vi "Multi-nRF24-BME280-Logger-v1.0.0.vi"() -> ()   [LabVIEW 2018]
uses:
  Program Files (x86)/National Instruments/LabVIEW 2018/examples/Instrument IO/Serial/support/Serial - XON-XOFF Characters.ctl
  Program Files (x86)/National Instruments/LabVIEW 2018/examples/Instrument IO/Serial/support/Serial - ASCII Characters.ctl
  Program Files (x86)/National Instruments/LabVIEW 2018/examples/Instrument IO/Serial/support/Serial - Settings.ctl
  <vilib>/Instr/_visa.llb/VISA Configure Serial Port (Instr).vi
panel:
  in  "Start Button":bool
  out "Log String":string
  in  "No. Of Sensor Modules":i32
  out "error out":errorcluster
  in  "VISA resource name":refnum<visa-resource-name>="COM1"
  out "Response":string
  in  "Stop":bool
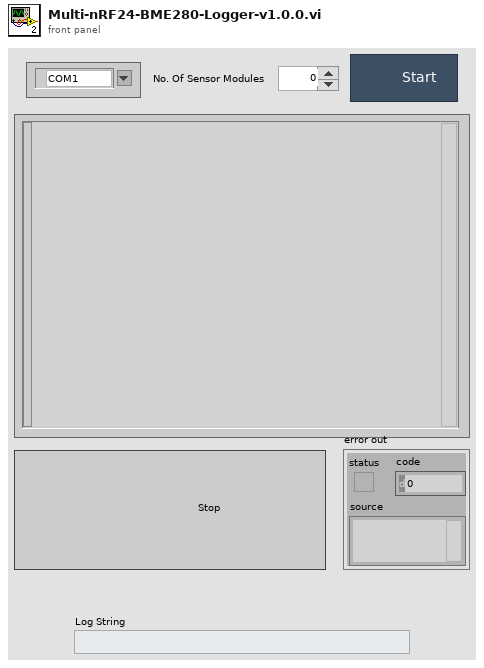
[diagram p1: front panel]
types:
  T1 = typedef "Serial - Settings.ctl" = cluster{"baud rate":u32, "data bits":u16, "parity":enum16{"None", "Odd", "Even", "Mark", "Space"}, "stop bits":u16, "flow control":u16}
  T2 = typedef "Serial - XON-XOFF Characters.ctl" = cluster{"XON":T3, "XOFF":T3}
  T3 = typedef "Serial - ASCII Characters.ctl" = enum16{"NUL", "SOH", "STX", "ETX", "EOT", "ENQ", "ACK", "BEL", "BS", "HT", "LF", "VT", "FF", "CR", "SO", "SI", "DLE", "DC1", "DC2", "DC3", "DC4", "NAK", "SYN", "ETB", "CAN", "EM", "SUB", "ESC", "FS", "GS", "RS", "US", "SP", "!", "\"", "#", "$", "%", "&", "'", "(", ")", "*", "+", ",", "- (-)", ".", "/", "0", "1", "2", "3", "4", "5", "6", "7", "8", "9", ":", ";", "<", "=", ">", "?", "@", "A", "B", "C", "D", "E", "F", "G", "H", "I", "J", "K", "L", "M", "N", "O", "P", "Q", "R", "S", "T", "U", "V", "W", "X", "Y", "Z", "[", "\\", "]", "^", "_", "`", "a", "b", "c", "d", "e", "f", "g", "h", "i", "j", "k", "l", "m", "n", "o", "p", "q", "r", "s", "t", "u", "v", "w", "x", "y", "z", "{", "|", "}", "~"}
  T4 = enum16{"open", "replace", "create", "open or create", "replace or create", "replace or create with confirmation"}
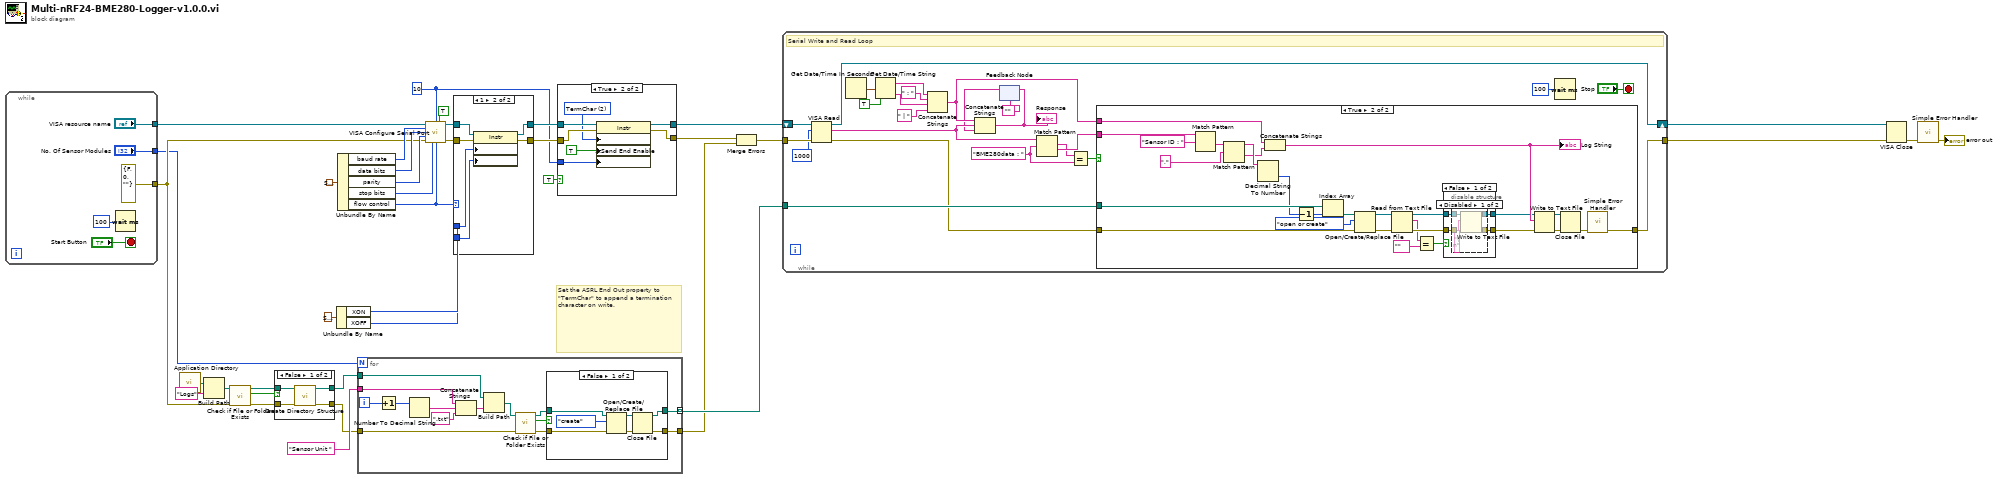
[diagram p0: block diagram]
diagram:
  w8 = u8 10 ("Termination Character")
  # "Set the ASRL End Out property to \"TermChar\" to append a termination character on write."
  n1 = while {
    tunnel: ["No. Of Sensor Modules"] -> w1
    tunnel: ["VISA resource name"] -> w28
    tunnel: [errorcluster {"status"=FALSE, "code"=0, "source"=""} ("error in (no error)")] -> w6
    stop <- "Start Button" stop-if-true
    n2 = Wait (ms)(milliseconds to wait=u32 100) -> ()  [unwired: 1 out]
  }
  n3 = call <vilib>:"Application Directory.vi"() -> ("Application Directory"=w29:path)
  n4 = Build Path(base path=w29, name or relative path="Logs") -> (appended path=w36:path)
  n5 = call <vilib>:"Check if File or Folder Exists.vi"("error in (no error)"=w6, "path"=w36) -> ("error out"=w32:errorcluster, "file or folder exists?"=w34:bool, "dup path"=w33:path)  [unwired: 7 in]
  n6 = case shown="False" w34 {
    tunnel: w33 -> [w46 w48]
    tunnel: w32 -> [w45 w47]
    tunnel: [w44 w48] -> w31
    tunnel: [w43 w47] -> w30
    frame False {
      n7 = call "Create Directory Structure.vi"("error in(no error)"=w45, "Dir Path In"=w46) -> ("error out"=w43:errorcluster, "Dir Path Out"=w44:path)  [unwired: 8 in]
    }
    frame True {
    }
  }
  n8 = Unbundle By Name(T2 {"XON"=enum."DC1", "XOFF"=enum."DC3"} ("XON/XOFF Characters")) -> ("XON"=w14:T3, "XOFF"=w13:T3)
  n9 = Unbundle By Name(T1 {"baud rate"=115200, "data bits"=8, "parity"=enum."None", "stop bits"=10, "flow control"=0} ("Serial Settings")) -> ("baud rate"=w21:u32, "data bits"=w22:u16, "parity"=w23:enum16{"None", "Odd", "Even", "Mark", "Space"}, "stop bits"=w24:u16, "flow control"=w15:u16)
  n10 = for {
    N: w1 -> [_]
    tunnel: "Sensor Unit " ("name or relative path") -> [w60]
    tunnel: w31 -> [w56]
    tunnel: w30 -> [w54]
    tunnel: [w50] -> w5 mode=indexing
    tunnel: [w49] -> w4
    i -> [w62]
    n11 = Increment(x=w62) -> (x+1=w61:i32)
    n12 = Number To Decimal String(number=w61) -> (decimal integer string=w59:string)  [unwired: 1 in]
    n13 = Concatenate Strings(w60, w59, ".txt" ("string")) -> (w57:string)
    n14 = Build Path(base path=w56, name or relative path=w57) -> (appended path=w55:path)
    n15 = call <vilib>:"Check if File or Folder Exists.vi"("error in (no error)"=w54, "path"=w55) -> ("error out"=w51:errorcluster, "file or folder exists?"=w53:bool, "dup path"=w52:path)  [unwired: 7 in]
    n16 = case shown="False" w53 {
      tunnel: w52 -> [w67 w71]
      tunnel: w51 -> [w68 w70]
      tunnel: [w65 w71] -> w50
      tunnel: [w63 w70] -> w49
      frame False {
        n17 = Open/Create/Replace File(file path (use dialog)=w67, error in=w68, operation (0:open)=T4."create") -> (refnum out=w66:refnum<file>, error out=w64:errorcluster)  [unwired: 3 in, 1 out]
        n18 = Close File(refnum=w66, error in=w64) -> (path=w65:path, error out=w63:errorcluster)
      }
      frame True {
      }
    }
  }
  n19 = call-poly "VISA Configure Serial Port"("VISA resource name"=w28, "termination char\n(0xA = '\\n' = LF)"=w8, "Enable Termination\nChar (T)"=TRUE ("End Read on Termination Character?"), "baud rate (9600)"=w21, "data bits (8)"=w22, "parity (0:none)"=w23, "error in (no error)"=w6, "stop bits (10: 1 bit)"=w24, "flow control (0:none)"=w15) -> ("VISA resource name out"=w25:refnum<visa-resource-name>, "error out"=w26:errorcluster)  [unwired: 1 in, 4 out]
  n20 = case shown="1" w15 {
    tunnel: [w72 w79] -> w12
    tunnel: [w73 w78] -> w11
    tunnel: w26 -> [w72 w77]
    tunnel: w25 -> [w73 w76]
    tunnel: w14 -> [_ w75]
    tunnel: w13 -> [_ w74]
    frame Default {
    }
    frame 1 {
      n21 = property class="Instr"(reference=w76, error in=w77, "Serial Settings:Flow Control XON Character"=w75, "Serial Settings:Flow Control XOFF Character"=w74) -> (reference out=w78:refnum<visa-resource-name>, error out=w79:errorcluster)
    }
  }
  n22 = case shown="True" TRUE ("End Write on Termination Character?") {
    tunnel: w11 -> [w80 w88]
    tunnel: w12 -> [w81 w87]
    tunnel: [w80 w86] -> w10
    tunnel: [w81 w85] -> w3
    tunnel: w8 -> [_ w83]
    frame False {
    }
    frame True {
      w84 = u16 2 items=["None", "LastBit", "TermChar", "Break"] ("Serial Settings:Serial End Mode for Writes")
      n23 = property class="Instr"(reference=w88, error in=w87, "Serial Settings:End Mode for Writes"=w84, "Message Based Settings:Send End Enable"=TRUE, "Message Based Settings:Termination Character"=w83) -> (reference out=w86:refnum<visa-resource-name>, error out=w85:errorcluster)
    }
  }
  n24 = Merge Errors(w3, w4) -> (w2:errorcluster)
  n25 = while {
    shift-right: [w107] -> w16
    shift-left: w10 -> [w112]
    tunnel: w2 -> [w111]
    tunnel: [w90] -> w17
    tunnel: w5 -> [w92]
    stop <- "Stop" stop-if-true
    w94 = "BME280data : "
    # "Serial Write and Read Loop"
    n26 = VISA Read(VISA resource name=w112, byte count=u32 1000 ("Read Count"), error in (no error)=w111) -> (VISA resource name out=w107:refnum<visa-resource-name>, read buffer=w93:string, error out=w91:errorcluster)  [unwired: 1 out]
    n27 = Get Date/Time In Seconds() -> (seconds since 1Jan1904=w103:timestamp)
    n28 = Get Date/Time String(seconds (now)=w103, want seconds? (F)=TRUE) -> (date string=w104:string, time string=w102:string)  [unwired: 1 in]
    n29 = Concatenate Strings(w104, " : " ("string"), w102, " | " ("string")) -> (w105:string)
    n30 = feedback #1("") -> (w89:string)
    n31 = Concatenate Strings(w105, w93, w89) -> (w106:string)
    "Response" <- w106
    n32 = feedback-in #1(w106) -> ()
    n33 = Match Pattern(string=w93, regular expression=w94) -> (match substring=w99:string, after substring=w101:string)  [unwired: 1 in, 2 out]
    n34 = Equal?(x=w99, y=w94) -> (x = y?=w100:bool)
    n35 = case shown="True" w100 {
      tunnel: w101 -> [_ w140]
      tunnel: w105 -> [_ w133]
      tunnel: w92 -> [_ w135]
      tunnel: w91 -> [w113 w125]
      tunnel: [w113 w124] -> w90
      frame False {
      }
      frame True {
        n36 = Match Pattern(string=w140, regular expression="Sensor ID : ") -> (after substring=w138:string)  [unwired: 1 in, 3 out]
        n37 = Match Pattern(string=w138, regular expression=",") -> (before substring=w136:string, after substring=w132:string)  [unwired: 1 in, 2 out]
        n38 = Decimal String To Number(string=w136) -> (number=w123:i32)  [unwired: 2 in, 1 out]
        n39 = Concatenate Strings(w133, w132) -> (w126:string)
        "Log String" <- w126
        n40 = Decrement(x=w123) -> (x-1=w134:i32)
        n41 = Index Array(array=w135, index=w134) -> (element=w127:path)
        n42 = Open/Create/Replace File(file path (use dialog)=w127, error in=w125, operation (0:open)=T4."open or create") -> (refnum out=w117:refnum<file>, error out=w116:errorcluster)  [unwired: 3 in, 1 out]
        n43 = Read from Text File(file (use dialog)=w117, error in=w116) -> (refnum out=w122:refnum<file>, text=w120:string, error out=w121:errorcluster)  [unwired: 2 in, 1 out]
        n44 = Equal?(x=w120, y="" ("string")) -> (x = y?=w119:bool)
        n45 = case shown="False" w119 {
          tunnel: w122 -> [w144 w153]
          tunnel: [w143 w153] -> w115
          tunnel: w121 -> [w142 w152]
          tunnel: [w141 w152] -> w114
          frame False {
            n46 = disable-structure shown="Disabled" {
              disable-tunnel: w144 -> [w148 w151]
              disable-tunnel: [w147 w151] -> w143
              disable-tunnel: w142 -> [w146 w150]
              disable-tunnel: [w145 w150] -> w141
              frame Disabled {
                n47 = Write to Text File(file (use dialog)=w148, text="\n", error in=w146) -> (refnum out=w147:refnum<file>, error out=w145:errorcluster)  [unwired: 1 in, 1 out]
              }
              frame Enabled {
              }
            }
          }
          frame True {
          }
        }
        n48 = Write to Text File(file (use dialog)=w115, text=w126, error in=w114) -> (refnum out=w130:refnum<file>, error out=w131:errorcluster)  [unwired: 1 in, 1 out]
        n49 = Close File(refnum=w130, error in=w131) -> (error out=w128:errorcluster)  [unwired: 1 out]
        n50 = call <vilib>:"Simple Error Handler.vi"("error in (no error)"=w128) -> ("error out"=w124:errorcluster)  [unwired: 4 in, 4 out]
      }
    }
    n51 = Wait (ms)(milliseconds to wait=u32 100) -> ()  [unwired: 1 out]
  }
  n52 = VISA Close(VISA resource name=w16, error in (no error)=w17) -> (error out=w18:errorcluster)
  n53 = call <vilib>:"Simple Error Handler.vi"("error in (no error)"=w18) -> ("error out"=→"error out":errorcluster)  [unwired: 1 in, 7 out]
